vi "report timing.vi"(9 "status reporting tags":T3, 10 "time data in":T1, 11 "engine tag bus":T2) -> (2 "time data out":T1, 3 "engine data out":T2)   [LabVIEW 2013, in "main engine.lvlib"]
uses:
  main engine/main engine.lvlib
  status reporting data.ctl
  <vilib>/NI/Tag Bus/table/data table.ctl
  time information.ctl
  <vilib>/NI/Tag Bus/table/data polymorphs/write one/write Boolean.vi
  <vilib>/NI/Tag Bus/table/data polymorphs/write one/write U32.vi
  <vilib>/NI/Tag Bus/table/data polymorphs/write one/write U64.vi
  <vilib>/NI/Tag Bus/table/data table.lvlib
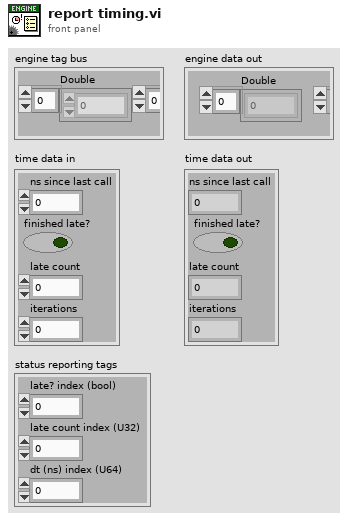
[diagram p1: front panel]
types:
  T1 = typedef "main engine.lvlib/time information.ctl" = cluster{"ns since last call":u64, "finished late?":bool, "late count":u32, "iterations":u64}
  T2 = typedef "tag bus.lvlib/data table.lvlib/data table.ctl" = cluster{"Double":dbl[], "Single":sgl[], "I64":i64[], "I32":i32[], "I16":i16[], "I8":i8[], "U64":u64[], "U32":u32[], "U16":u16[], "U8":u8[], "Boolean":bool[], "String":string[], "Array of Double":cluster{"DBL Array":dbl[]}[], "Array of Single":cluster{"SGL Array":sgl[]}[], "Array of I64":cluster{"I64 Array":i64[]}[], "Array of I32":cluster{"I32 Array":i32[]}[], "Array of I16":cluster{"I16 Array":i16[]}[], "Array of I8":cluster{"I8 Array":i8[]}[], "Array of U64":cluster{"U64 Array":u64[]}[], "Array of U32":cluster{"U32 Array":u32[]}[], "Array of U16":cluster{"U16 Array":u16[]}[], "Array of U8":cluster{"U8 Array":u8[]}[], "Array of Boolean":cluster{"Boolean Array":bool[]}[], "Array of String":cluster{"String Array":string[]}[]}
  T3 = typedef "main engine.lvlib/status reporting data.ctl" = cluster{"late? index (bool)":i32, "late count index (U32)":i32, "dt (ns) index (U64)":i32}
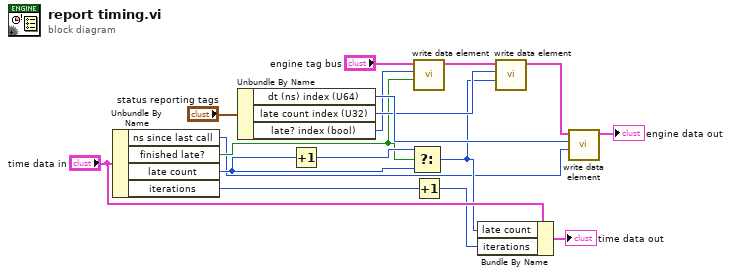
[diagram p0: block diagram]
diagram:
  n1 = Unbundle By Name("time data in") -> ("ns since last call"=w1:u64, "finished late?"=w2:bool, "late count"=w3:u32, "iterations"=w4:u64)
  n2 = Unbundle By Name("status reporting tags") -> ("dt (ns) index (U64)"=w17:i32, "late count index (U32)"=w16:i32, "late? index (bool)"=w15:i32)
  n3 = Increment(x=w3) -> (x+1=w9:u32)
  n4 = Select(t=w9, s=w2, f=w3) -> (s? t:f=w6:u32)
  n5 = call-poly <vilib>:"write data element.vi"("value"=w2, "index"=w15, "data table in"="engine tag bus") -> ("data table out"=w11:T2)  [unwired: 8 in]
  n6 = Increment(x=w4) -> (x+1=w5:u64)
  n7 = Bundle By Name(cluster="time data in", "late count"=w6, "iterations"=w5) -> (→"time data out":T1)
  n8 = call-poly <vilib>:"write data element.vi"("value"=w6, "index"=w16, "data table in"=w11) -> ("data table out"=w10:T2)  [unwired: 8 in]
  n9 = call-poly <vilib>:"write data element.vi"("value"=w1, "index"=w17, "data table in"=w10) -> ("data table out"=→"engine data out":T2)  [unwired: 8 in]
